vi "Remove_IconEd_Data.vi"(8 "error in (no error)":errorcluster, 10 "saveLevel":u32, 11 "Build in":refnum<class "AB_SourceDistribution.lvclass">) -> (0 "error out":errorcluster, 2 "remove":bool, 3 "Build out":refnum<class "AB_SourceDistribution.lvclass">)   [LabVIEW 2020, in "AB_SourceDistribution.lvclass"]
uses:
  <vilib>/AppBuilder/AB_Classes/SourceDistribution/AB_SourceDistribution.lvclass
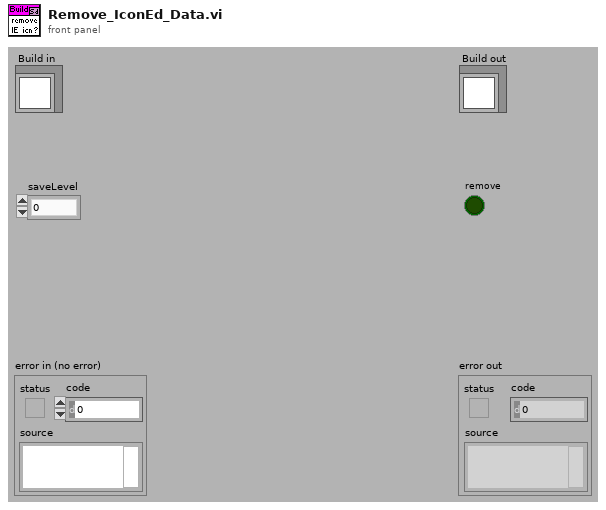
[diagram p1: front panel]
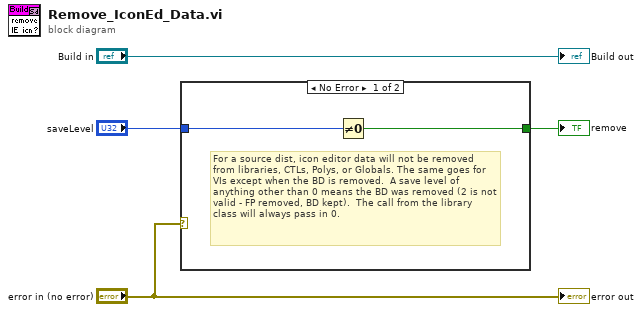
[diagram p0: block diagram]
diagram:
  n1 = case shown="No Error" "error in (no error)" {
    tunnel: "saveLevel" -> [w6 _]
    tunnel: [w5 _] -> w1
    frame No Error {
      # "For a source dist, icon editor data will not be removed from libraries, CTLs, Polys, or Globals. The same goes for VIs except when the BD is removed.  A save level of anything other than 0 means the BD was removed (2 is not valid - FP removed, BD kept).  The call from the library class will always pass in 0."
      n2 = Not Equal To 0?(x=w6) -> (x != 0?=w5:bool)
    }
    frame Error {
    }
  }
  "remove" <- w1
  "error out" <- "error in (no error)"
  "Build out" <- "Build in"
